vi "MoAgSy_Visitor_travel.appendData2Variant.vi"(0 "initData":variant, 2 "destination":string, 5 "error in":errorcluster) -> (14 "dup initData":variant, 19 "error out":errorcluster)   [LabVIEW 2009, in "MoAgSy.lvlib" / "MoAgSy_Visitor_travel.lvclass"]
doc: "append init data\ndestination: agents travel destination"
uses:
  MoAgSy_Visitor_travel.lvclass
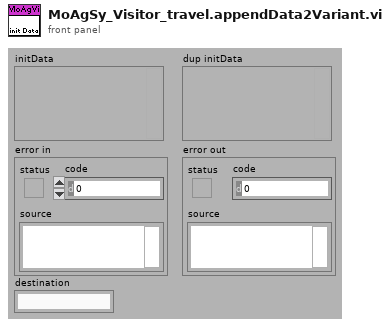
[diagram p1: front panel]
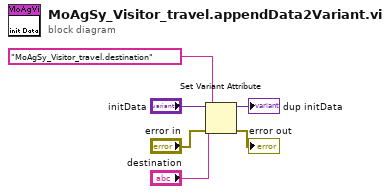
[diagram p0: block diagram]
diagram:
  n1 = Set Variant Attribute(Variant="initData", name="MoAgSy_Visitor_travel.destination", value="destination", error in="error in") -> (Variant out=→"dup initData":variant, error out=→"error out":errorcluster)  [unwired: 1 out]
